vi "ConfigTiming.vi"(8 "error in (no error)":errorcluster, 11 "PXI_MultiTrig in":refnum<class "PXI_MultiTrig.lvclass">) -> (0 "error out":errorcluster, 3 "PXI_MultiTrig out":refnum<class "PXI_MultiTrig.lvclass">)   [LabVIEW 2018, in "SyncPlugins.lvlib" / "PXI_MultiTrig.lvclass"]
uses:
  PXI_MultiTrig.lvclass
  X:/Projects/PMUCal/Modules/Sync/SyncPlugins/SyncPluginBase/SyncPluginBase.lvclass
  PXI_MultiTrig.lvclass/PXI_MultiTrig.ctl
  SyncPluginBase/SyncPluginBase.lvclass/SyncPluginBase.ctl
  Accessors/Read RefClkSource.vi
  Accessors/Read RefClkSession.vi
  Accessors/Read TimingHandle.vi
  Accessors/Write RefClkSession.vi
  Accessors/Write TimingSession.vi
  SyncPluginBase/Accessors/Write Initiated.vi
  <instrlib>/niSync/niSync.llb/niSync Create Clock (Frequency).vi
  <instrlib>/niSync/niSync.llb/niSync Initialize (IVI).vi
  <vilib>/Utility/error.llb/Error Cluster From Error Code.vi
  <vilib>/ErrorRing/Error Ring.xnode
panel:
  out "Retries":i32=2
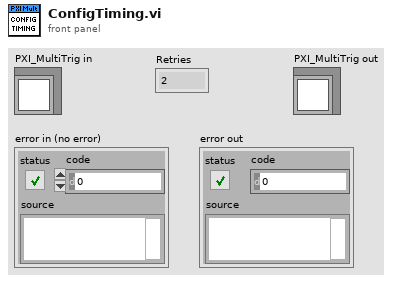
[diagram p1: front panel]
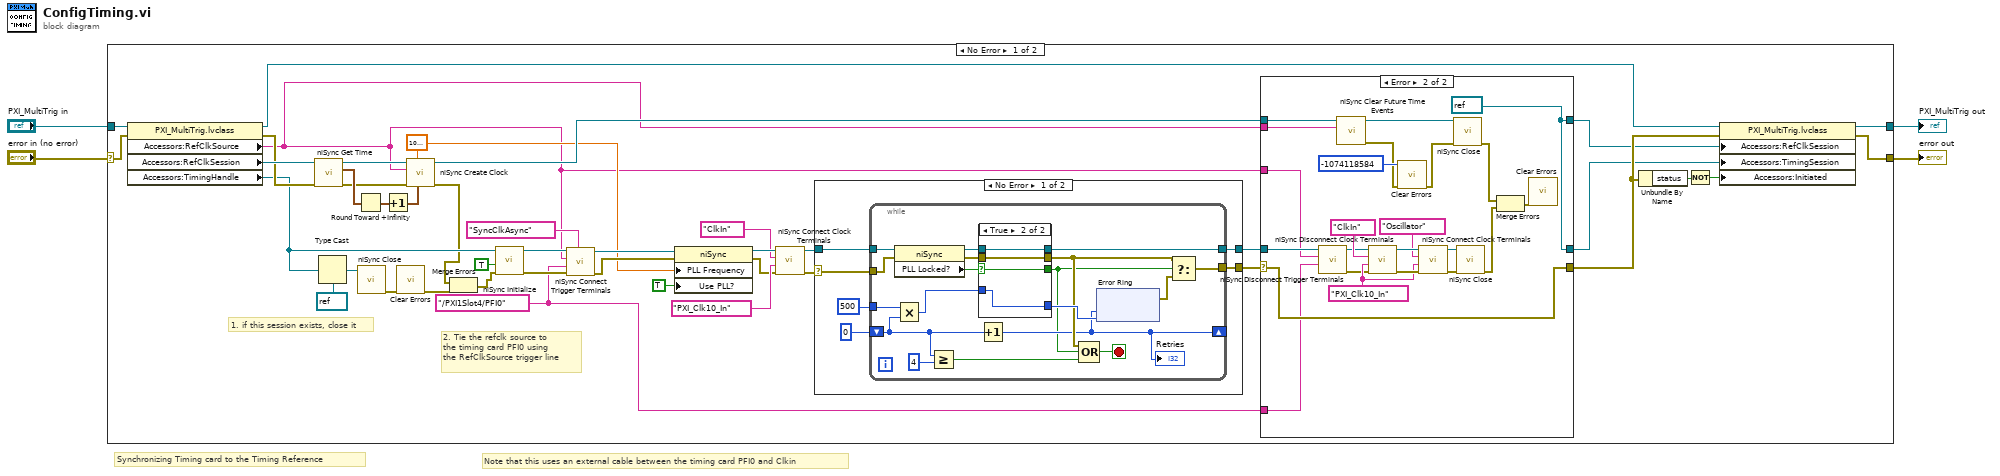
[diagram p0: block diagram]
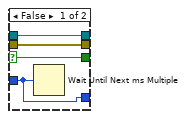
[diagram p3: hidden frame]
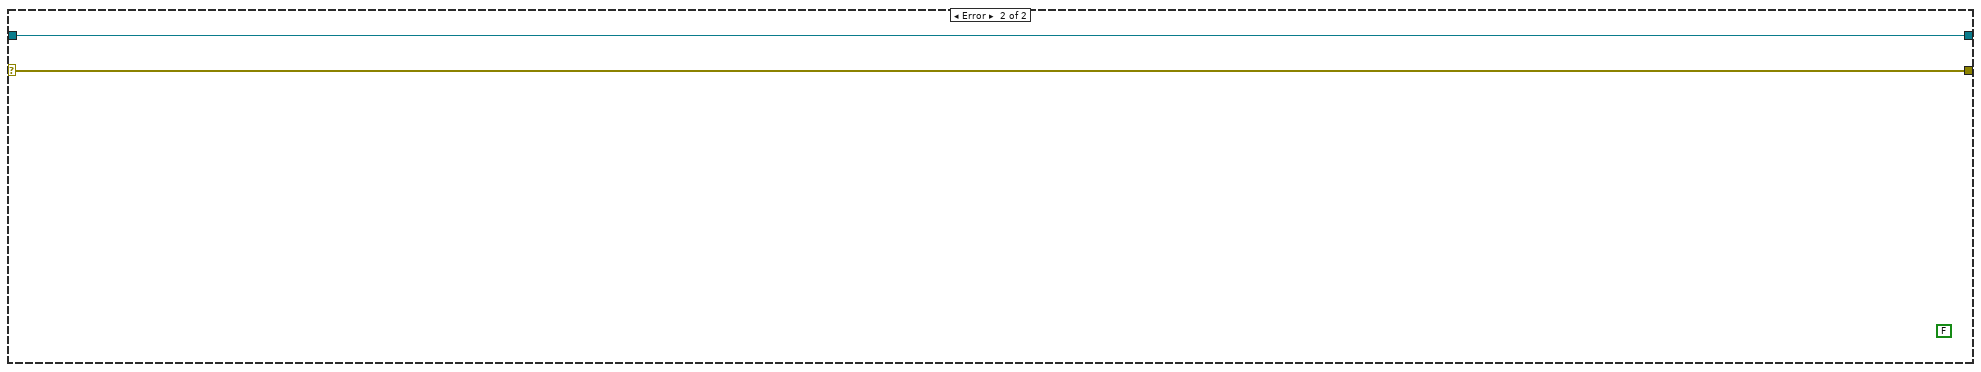
[diagram p5: hidden frame]
diagram:
  # "Note that this uses an external cable between the timing card PFI0 and Clkin"
  # "Synchronizing Timing card to the Timing Reference"
  n1 = case shown="No Error" "error in (no error)" {
    selector: "error in (no error)" -> [w43 w116]
    tunnel: [w47 w116] -> w4
    tunnel: [w44 w117] -> w3
    tunnel: "PXI_MultiTrig in" -> [w42 w117]
    frame No Error {
      w5 = "/PXI1Slot4/PFI0" ("destination terminal")
      w7 = 1000000.0 ("frequency")
      # "2. Tie the refclk source to\nthe timing card PFI0 using\nthe RefClkSource trigger line"
      # "1. if this session exists, close it"
      n2 = property class="PXI_MultiTrig.lvclass"(reference=w42, error in=w43) -> (reference out=w41:refnum<class "PXI_MultiTrig.lvclass">, error out=w32:errorcluster, "Accessors:RefClkSource"=w6:string, "Accessors:RefClkSession"=w35:refnum<k15>, "Accessors:TimingHandle"=w11:refnum<k15>)
      n3 = call <instrlib>:"niSync Get Time.vi"("error in (no error)"=w32, "instrument handle"=w35) -> ("error out"=w19:errorcluster, "time"=w22:timestamp, "instrument handle out"=w20:refnum<k15>)  [unwired: 5 in]
      n4 = Type Cast(type=refnum<k15> refnum ("instrument handle"), x=w11) -> (*(type *) &x=w13:refnum<k15>)
      n5 = Round Toward +Infinity(x=w22) -> (ceil(x): smallest int >= x=w21:timestamp)
      n6 = call <instrlib>:"niSync Close.vi"("instrument handle"=w13) -> ("error out"=w12:errorcluster)  [unwired: 10 in]
      n7 = Increment(x=w21) -> (x+1=w18:timestamp)
      n8 = call <vilib>:"Clear Errors.vi"("error in (no error)"=w12) -> ("error out"=w10:errorcluster)  [unwired: 5 in, 1 out]
      n9 = call-poly <instrlib>:"niSync Create Clock.vi"("start time"=w18, "frequency"=w7, "error in (no error)"=w19, "terminal"=w6, "instrument handle"=w20) -> ("error out"=w9:errorcluster, "instrument handle out"=w27:refnum<k15>)  [unwired: 3 in, 2 out]
      n10 = Merge Errors(w9, w10) -> (w8:errorcluster)
      n11 = call-poly <instrlib>:"niSync Initialize.vi"("error in (no error)"=w8, "reset device (F)"=TRUE ("id query"), "resource name"=w11) -> ("error out"=w15:errorcluster, "instrument handle out"=w17:refnum<k15>)  [unwired: 7 in]
      n12 = call <instrlib>:"niSync Connect Trigger Terminals.vi"("synchronization clock"="SyncClkAsync", "error in (no error)"=w15, "destination terminal"=w5, "source terminal"=w6, "instrument handle"=w17) -> ("error out"=w33:errorcluster, "instrument handle out"=w34:refnum<k15>)  [unwired: 5 in]
      n13 = property class="niSync"(reference=w34, error in=w33, "PLL Frequency"=w7, "Use PLL?"=TRUE ("Clk Properties:Use PLL?")) -> (reference out=w40:refnum<k15>, error out=w37:errorcluster)
      n14 = call <instrlib>:"niSync Connect Clock Terminals.vi"("error in (no error)"=w37, "destination terminal"="PXI_Clk10_In", "source terminal"="ClkIn", "instrument handle"=w40) -> ("error out"=w30:errorcluster, "instrument handle out"=w31:refnum<k15>)  [unwired: 6 in]
      n15 = case shown="No Error" w30 {
        selector: w30 -> [w79 w114]
        tunnel: w31 -> [w78 w115]
        tunnel: [w75 w114] -> w29
        tunnel: [w74 w115] -> w28
        frame No Error {
          n16 = while {
            tunnel: w79 -> [w94]
            tunnel: w78 -> [w93]
            shift-right: [w81] -> _
            shift-left: 0 -> [w88]
            tunnel: u32 500 ("PllWait") -> [w95]
            tunnel: [w83] -> w75
            tunnel: [w82] -> w74
            stop <- w89 stop-if-true
            n17 = property class="niSync"(reference=w93, error in=w94) -> (reference out=w91:refnum<k15>, error out=w92:errorcluster, "PLL Locked?"=w90:bool)
            n18 = Multiply(x=w95, y=w88) -> (x*y=w87:u32)
            n19 = Greater Or Equal?(x=w88, y=4) -> (x >= y?=w96:bool)
            n20 = case shown="True" w90 {
              selector: w90 -> [w109 w111]
              tunnel: w92 -> [w108 w112]
              tunnel: w91 -> [w107 w113]
              tunnel: [w107 w113] -> w82
              tunnel: [w108 w112] -> w85
              tunnel: [w109 w111] -> w80
              tunnel: w87 -> [w106 w110]
              tunnel: [w106 w110] -> w86
              frame False {
                n21 = Wait Until Next ms Multiple(millisecond multiple=w106) -> ()  [unwired: 1 out]
              }
              frame True {
              }
            }
            n22 = Increment(x=w88) -> (x+1=w81:i32)
            "Retries" <- w81
            n23 = Compound Arithmetic op=OR(w85, w80, w96) -> (w89:bool)
            n24 = xnode "Error Ring"("parameter 0"=w81, "parameter 1"=w86) -> ("error out"=w84:errorcluster)
            n25 = Select(t=w85, s=w80, f=w84) -> (s? t:f=w83:errorcluster)
          }
        }
        frame Error {
        }
      }
      n26 = case shown="Error" w29 {
        selector: w29 -> [w50 w61]
        tunnel: w28 -> [w48 w55]
        tunnel: w27 -> [w49 w73]
        tunnel: w6 -> [_ w72]
        tunnel: [w50 w61] -> w26
        tunnel: [w49 w69] -> w25
        tunnel: [w48 w69] -> w24
        tunnel: w6 -> [_ w52]
        tunnel: w5 -> [_ w51]
        frame No Error {
        }
        frame Error {
          w65 = "PXI_Clk10_In" ("destination terminal")
          w69 = refnum<k15> refnum ("instrument handle out")
          n27 = call <instrlib>:"niSync Disconnect Trigger Terminals.vi"("destination terminal"=w51, "source terminal"=w52, "instrument handle"=w55) -> ("error out"=w53:errorcluster, "instrument handle out"=w54:refnum<k15>)  [unwired: 7 in]
          n28 = call <instrlib>:"niSync Clear Future Time Events.vi"("terminal"=w72, "instrument handle"=w73) -> ("error out"=w56:errorcluster, "instrument handle out"=w71:refnum<k15>)  [unwired: 7 in]
          n29 = call <instrlib>:"niSync Disconnect Clock Terminals.vi"("error in (no error)"=w53, "destination terminal"=w65, "source terminal"="ClkIn", "instrument handle"=w54) -> ("error out"=w67:errorcluster, "instrument handle out"=w66:refnum<k15>)  [unwired: 6 in]
          n30 = call <vilib>:"Clear Errors.vi"("error in (no error)"=w56, "specific error code to clear (0: all)"=-1074118584) -> ("error out"=w70:errorcluster)  [unwired: 4 in, 1 out]
          n31 = call <instrlib>:"niSync Connect Clock Terminals.vi"("error in (no error)"=w67, "destination terminal"=w65, "source terminal"="Oscillator", "instrument handle"=w66) -> ("error out"=w63:errorcluster, "instrument handle out"=w62:refnum<k15>)  [unwired: 6 in]
          n32 = call <instrlib>:"niSync Close.vi"("error in (no error)"=w70, "instrument handle"=w71) -> ("error out"=w59:errorcluster)  [unwired: 9 in]
          n33 = call <instrlib>:"niSync Close.vi"("error in (no error)"=w63, "instrument handle"=w62) -> ("error out"=w60:errorcluster)  [unwired: 9 in]
          n34 = Merge Errors(w59, w60) -> (w58:errorcluster)
          n35 = call <vilib>:"Clear Errors.vi"("error in (no error)"=w58) -> ()  [unwired: 5 in, 2 out]
        }
      }
      n36 = Unbundle By Name(w26) -> ("status"=w45:bool)
      n37 = Not(x=w45) -> (.not. x?=w46:bool)
      n38 = property class="PXI_MultiTrig.lvclass"(reference=w41, error in=w26, "Accessors:RefClkSession"=w25, "Accessors:TimingSession"=w24, "Accessors:Initiated"=w46) -> (reference out=w44:refnum<class "PXI_MultiTrig.lvclass">, error out=w47:errorcluster)
    }
    frame Error {
      (unwired) FALSE
    }
  }
  "error out" <- w4
  "PXI_MultiTrig out" <- w3
